vi "manipulator_loop.vi"(5 "error in":errorcluster, 8 "Micron config":T1) -> (0 "error out":errorcluster)   [LabVIEW 2014]
uses:
  initialization/micron_config.ctl
  squiggle/Host/i2c_interface.ctl
  squiggle/Host/fpga_reference.ctl
  testing/Micron params.ctl
  testing/stimulus.ctl
  testing/injection_point.ctl
  filtering/goal_loop_parms.ctl
  testing/mode_conrols.ctl
  testing/manipulator_cal.ctl
  asap/labview/testing/probe_calibration.ctl
  host/network_params.ctl
  cancellation/sq_control_params.ctl
  cancellation/decoupled_gain.ctl
  cancellation/estimation_controls.ctl
  <vilib>/Platform/TimedLoop/XDataNode/timing_clust.ctl
  <vilib>/Platform/TimedLoop/XDataNode/nitl_modes.ctl
  <vilib>/Platform/TimedLoop/XDataNode/wakeup.ctl
  <vilib>/DAQmx/read.llb/DAQmx Read (Digital 1D Bool 1Chan 1Samp).vi
  <vilib>/DAQmx/read.llb/DAQmx Read (Analog 1D DBL NChan 1Samp).vi
  <vilib>/Platform/TimedLoop/XDataNode/XDataNode.xnode
  <vilib>/NI_Real-Time Target Support.lvlib
  <vilib>/Platform/TimedLoop/XDataNode/XDNodeRunTimeDep.lvlib
panel:
  in  "Times late":i32
  out "Mean times (uS)":dbl[](array[numeric]) format="%#.1f"
  in  "Profile iterations":i32=60000
  out "total time histogram":T4(graph)
  out "cumulative times (uS)":dbl[][](graph)
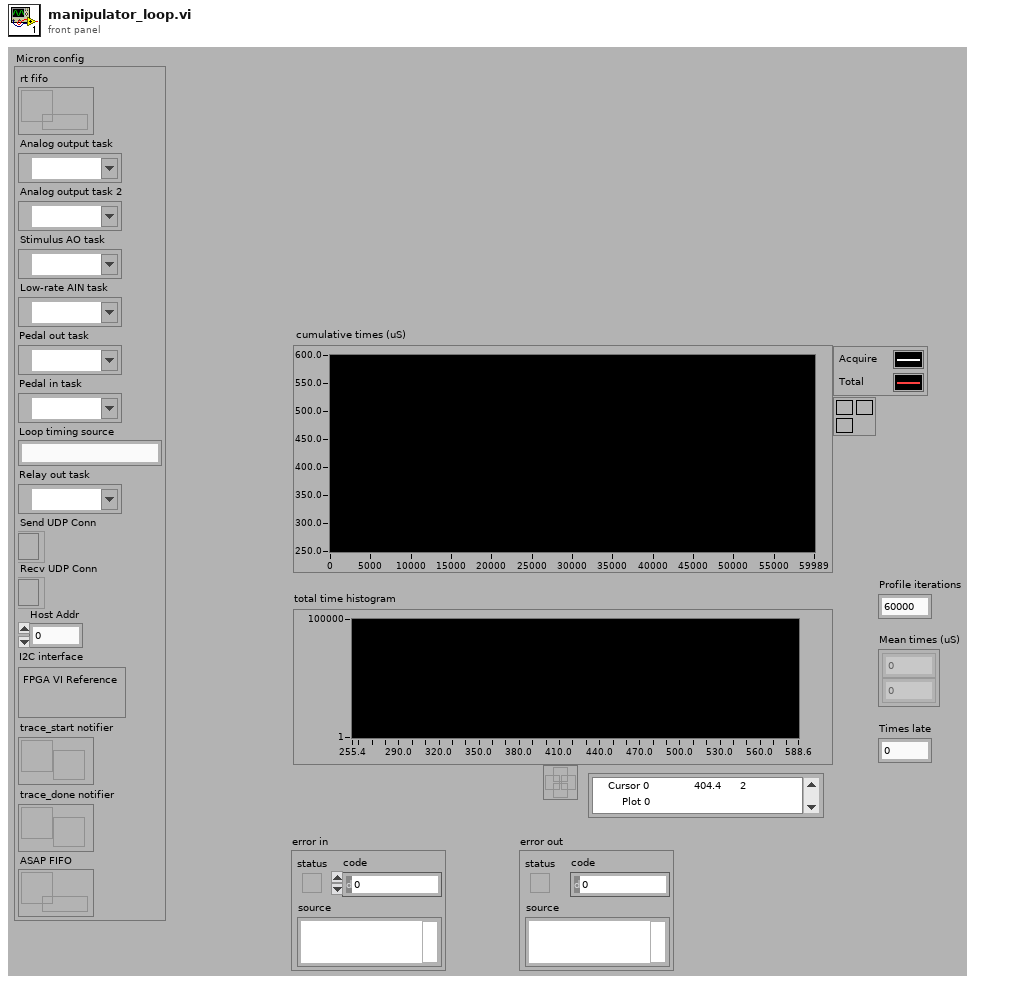
[diagram p1: front panel]
types:
  T1 = typedef "micron_config.ctl" = cluster{"rt fifo":refnum<k33>, "Analog output task":refnum<k21>, "Analog output task 2":refnum<k21>, "Stimulus AO task":refnum<k21>, "Low-rate AIN task":refnum<k21>, "Pedal out task":refnum<k21>, "Pedal in task":refnum<k21>, "Loop timing source":string, "Relay out task":refnum<k21>, "Send UDP Conn":refnum<k16>, "Recv UDP Conn":refnum<k16>, "Host Addr":u32, "I2C interface":T2, "trace_start notifier":refnum<notifier>, "trace_done notifier":refnum<notifier>, "ASAP FIFO":refnum<k33>}
  T2 = typedef "i2c_interface.ctl" = cluster{"FPGA VI Reference":T3}
  T3 = typedef "fpga_reference.ctl" = refnum<k20>
  T4 = cluster{"X Values":dbl[], "Histogram: h(x)":i32[]}
  T5 = typedef "XDNodeRunTimeDep.lvlib/timing_clust.ctl" = cluster{"Expected End [f-1]":u64, "Actual End [f-1]":u64, "Finished Late? [f-1]":bool, "Expected End [i-1]":u64, "Actual End [i-1]":u64, "Finished Late? [i-1]":bool, "Expected Start [i]":u64, "Actual Start [i]":u64, "Expected Start [f]":u64, "Actual Start [f]":u64, "Source Name":string, "Structure Name":string, "Period":i64, "Deadline":i64, "Offset":i64, "Start":i64, "Priority":i32, "Timeout":i32, "Mode":T6, "Wakeup Reason":T7, "Error":errorcluster, "Source Type":string, "Secondary Source Type":string, "Global End Time":u64, "Global Start Time":u64, "Frame Duration":u64, "Iteration Duration":u64, "Assigned CPU":i32, "I/O Scan Engine Mode":u32}
  T6 = typedef "XDNodeRunTimeDep.lvlib/nitl_modes.ctl" = enum32{"No Change", "Process missed periods, maintain original phase", "Discard missed periods, maintain original phase", "Process missed periods, ignore original phase", "Discard missed periods, ignore original phase"}
  T7 = typedef "XDNodeRunTimeDep.lvlib/wakeup.ctl" = enum32{"Normal", "Aborted", "Asynchronous wakeup", "Timing source error", "Timed loop error", "Timeout"}
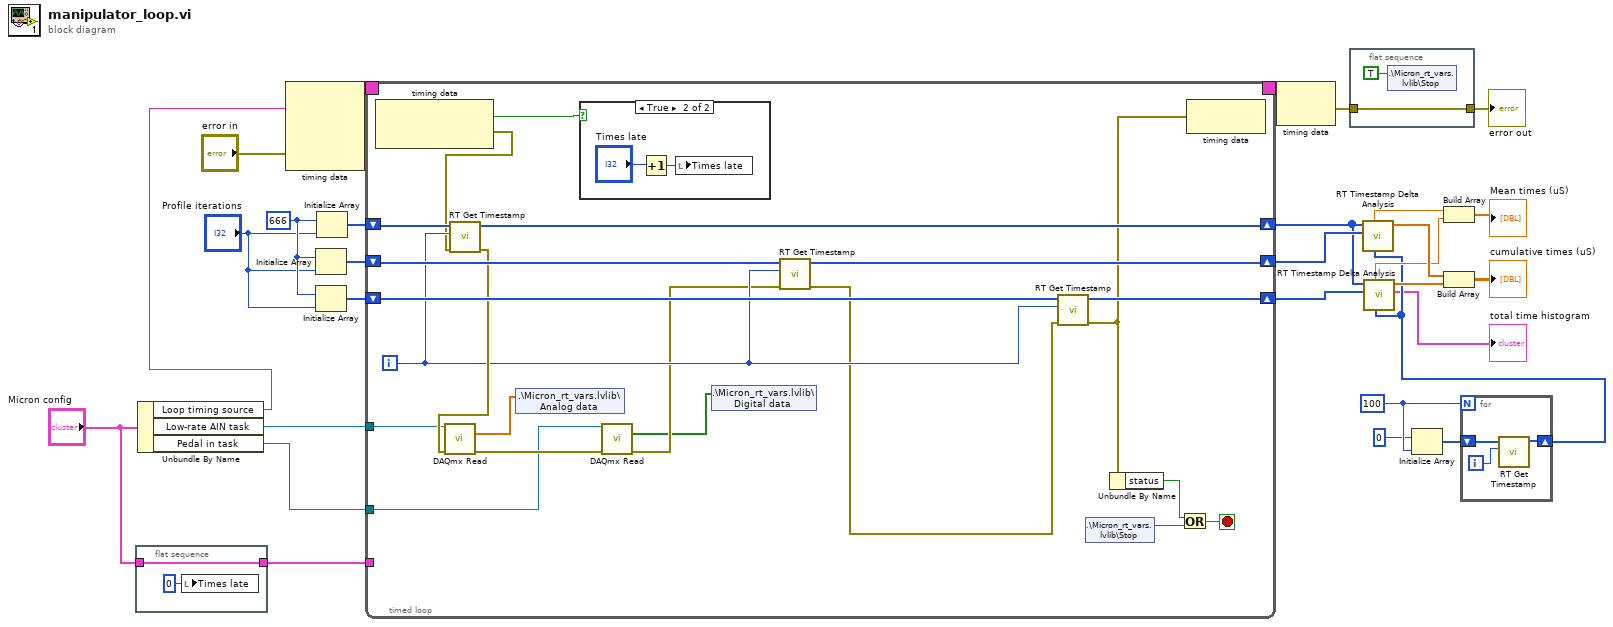
[diagram p0: block diagram]
diagram:
  w15 = u64 666 ("element")
  w22 = 100
  n1 = flat-sequence {
    tunnel: "Micron config" -> [w30]
    tunnel: [w30] -> w7
    frame #0 {
      n2 = local write "Times late"(0 ("Times late")) -> ()
    }
  }
  n3 = Unbundle By Name("Micron config") -> ("Loop timing source"=w6:string, "Low-rate AIN task"=w9:refnum<k21>, "Pedal in task"=w1:refnum<k21>)
  n4 = node-c288(w6, "error in") -> (w11:T5)  [unwired: 2 out]
  n5 = Initialize Array(w15, "Profile iterations") -> (w27:u64[])
  n6 = Initialize Array(w15, "Profile iterations") -> (w28:u64[])
  n7 = Initialize Array(w15, "Profile iterations") -> (w29:u64[])
  n8 = timed-loop "deterministic loop" {
    tunnel: w7 -> [_]
    shift-right: [w50] -> w19
    shift-left: w27 -> [w51]
    shift-right: [w48] -> w23
    shift-left: w28 -> [w49]
    shift-right: [w46] -> w13
    shift-left: w29 -> [w47]
    tunnel: w9 -> [w43]
    timing: w11 -> [_]
    timing-out: [_] -> w10
    tunnel: w1 -> [w33]
    i -> [w40]
    stop <- w45 stop-if-true
    n9 = node-c288() -> (w38:bool, w39:errorcluster)  [unwired: 1 out]
    n10 = call <vilib>:"RT Get Timestamp.vi"("error in (no error)"=w39, "iteration"=w40, "timestamp array in"=w47) -> ("error out"=w44:errorcluster, "timestamp array out"=w46:u64[])  [unwired: 7 out]
    n11 = call-poly <vilib>:"DAQmx Read.vi"("task/channels in"=w43, "error in"=w44) -> ("data"=w34:dbl[], "error out"=w37:errorcluster)  [unwired: 12 out]
    n12 = shared-variable ".\\Micron_rt_vars.lvlib\\Analog data"(w34) -> ()  [unwired: 2 out]
    n13 = case shown="True" w38 {
      frame False {
      }
      frame True {
        n14 = Increment(x="Times late") -> (x+1=w58:i32)
        n15 = local write "Times late"(w58) -> ()
      }
    }
    n16 = call-poly <vilib>:"DAQmx Read.vi"("task/channels in"=w33) -> ("data"=w32:bool[])  [unwired: 2 in, 12 out]
    n17 = shared-variable ".\\Micron_rt_vars.lvlib\\Digital data"(w32) -> ()  [unwired: 1 in, 1 out]
    n18 = call <vilib>:"RT Get Timestamp.vi"("error in (no error)"=w37, "iteration"=w40, "timestamp array in"=w51) -> ("error out"=w35:errorcluster, "timestamp array out"=w50:u64[])  [unwired: 7 out]
    n19 = call <vilib>:"RT Get Timestamp.vi"("error in (no error)"=w35, "iteration"=w40, "timestamp array in"=w49) -> ("error out"=w36:errorcluster, "timestamp array out"=w48:u64[])  [unwired: 7 out]
    n20 = shared-variable ".\\Micron_rt_vars.lvlib\\Stop"() -> (w41:bool)  [unwired: 2 out]
    n21 = Unbundle By Name(w36) -> ("status"=w42:bool)
    n22 = Or(x=w42, y=w41) -> (x .or. y?=w45:bool)
    n23 = node-c288(w36) -> ()  [unwired: 1 out]
  }
  n24 = node-c288(w10) -> (w3:errorcluster)
  n25 = flat-sequence {
    tunnel: w3 -> [w60]
    tunnel: [w60] -> w2
    frame #0 {
      n26 = shared-variable ".\\Micron_rt_vars.lvlib\\Stop"(TRUE ("Stop")) -> ()  [unwired: 2 out]
    }
  }
  n27 = Initialize Array(u64 0 ("element"), w22) -> (w21:u64[])
  n28 = for {
    N: w22 -> [_]
    shift-right: [w62] -> w12
    shift-left: w21 -> [w64]
    i -> [w63]
    n29 = call <vilib>:"RT Get Timestamp.vi"("iteration"=w63, "timestamp array in"=w64) -> ("timestamp array out"=w62:u64[])  [unwired: 1 in, 8 out]
  }
  n30 = call "RT Timestamp Delta Analysis.vi"("calibration array"=w12, "timestamp array 2"=w19, "timestamp array 1"=w13) -> ("execution times (uS)"=w24:dbl[], "mean time (uS)"=w18:dbl)  [unwired: 3 in, 4 out]
  n31 = call "RT Timestamp Delta Analysis.vi"("calibration array"=w12, "timestamp array 2"=w23, "timestamp array 1"=w13) -> ("execution histogram"=→"total time histogram":T4, "execution times (uS)"=w25:dbl[], "mean time (uS)"=w17:dbl)  [unwired: 3 in, 3 out]
  n32 = Build Array(w18, w17) -> (→"Mean times (uS)":dbl[])
  n33 = Build Array(w24, w25) -> (→"cumulative times (uS)":dbl[][])
  "error out" <- w2
